vi "ZK流程控制.vi"(7 "是否启用通讯通知":bool, 8 "error in (no error)":errorcluster, 10 "流程控制":T2, 11 "Slave ID":T1) -> (0 "error out":errorcluster)   [LabVIEW 2016, in "质控单元V4.lvlib"]
uses:
  <vilib>/Plasmionique/MB Master/MB_Master/MB_Master.lvclass
  <vilib>/Plasmionique/MB Master/MB Master.lvlib
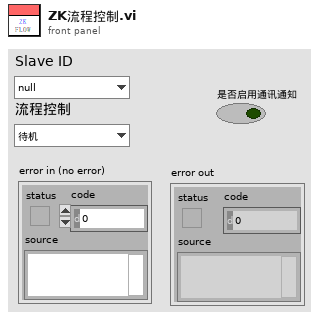
[diagram p1: front panel]
types:
  T1 = typedef "质控单元V4.lvlib/质控slave id.ctl" = enum16{"null", "氨氮", "总磷", "总氮", "CODMn", "CODCr", "氟化物", "挥发酚"}
  T2 = typedef "质控单元V4.lvlib/质控流程控制.ctl" = enum16{"待机", "启动进样流程", "启动加标流程", "启动排液流程", "启动水样润洗流程", "启动加标润洗流程", "停止流程"}
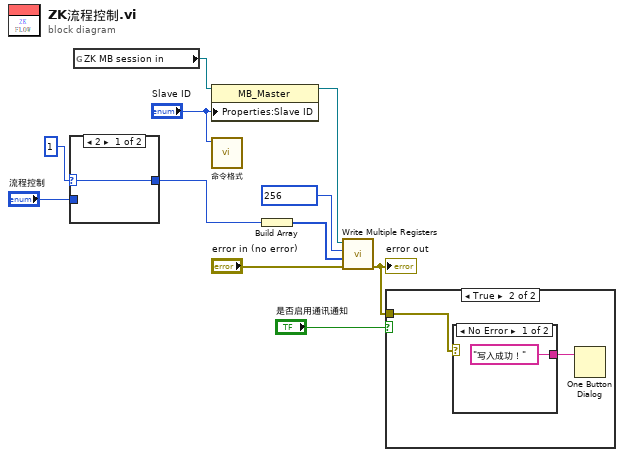
[diagram p0: block diagram]
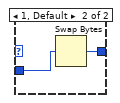
[diagram p2: hidden frame]
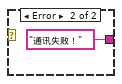
[diagram p4: hidden frame]
diagram:
  n1 = case shown="2" u16 1 ("命令格式") {
    selector: u16 1 ("命令格式") -> [w12 _]
    tunnel: "流程控制" -> [_ w14]
    tunnel: [w12 w13] -> w6
    frame 2 {
    }
    frame 1, Default {
      n2 = Swap Bytes(anything=w14) -> (byte swapped=w13:u16)
    }
  }
  n3 = global read "ZK非断电保存全局变量.vi" "ZK MB session in"() -> (w10:refnum<class "MB_Master.lvclass">)
  n4 = property class="MB_Master"(reference=w10, "Properties:Slave ID"="Slave ID") -> (reference out=w7:refnum<class "MB_Master.lvclass">)  [unwired: 1 in, 1 out]
  n5 = call "命令格式.vi"("站号"="Slave ID") -> ()  [unwired: 10 in, 1 out]
  n6 = Build Array(w6) -> (w5:u16[])
  n7 = call <vilib>:"Write Multiple Registers.vi"("error in (no error)"="error in (no error)", "values"=w5, "starting address"=u16 256, "MB session in"=w7) -> ("error out"=w3:errorcluster)  [unwired: 6 in, 1 out]
  "error out" <- w3
  n8 = case shown="True" "是否启用通讯通知" {
    tunnel: w3 -> [_ w16]
    frame False {
    }
    frame True {
      n9 = case shown="No Error" w16 {
        tunnel: ["写入成功！" "通讯失败！"] -> w15
        frame No Error {
        }
        frame Error {
        }
      }
      n10 = One Button Dialog(message=w15) -> ()  [unwired: 1 in, 1 out]
    }
  }
